vi "LWXPS_GetType.vi"(3 "LabVIEW error IN":errorcluster, 5 "XPS Reference IN":refnum<k24>) -> (0 "LabVIEW error OUT":errorcluster, 1 "Type":refnum<k24>, 2 "XPS Reference OUT":refnum<k24>)   [LabVIEW 2014]
uses:
  D:/XPSQ8_LabView_Library/Development/Source/Dll/Newport.XPS.CommandInterface.dll
  Dll/Newport.XPS.CommandInterface.dll
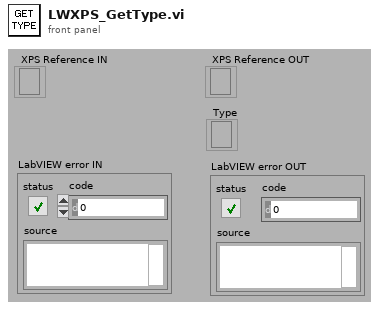
[diagram p1: front panel]
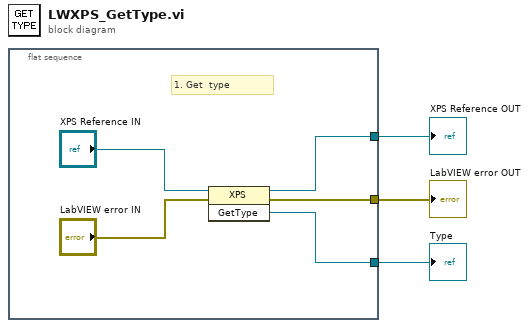
[diagram p0: block diagram]
diagram:
  n1 = flat-sequence {
    tunnel: [w7] -> w3
    tunnel: [w6] -> w2
    tunnel: [w4] -> w1
    frame #0 {
      # "1. Get  type"
      n2 = invoke class="XPS" method="GetType"(reference="XPS Reference IN", error in="LabVIEW error IN") -> (reference out=w7:refnum<k24>, error out=w6:errorcluster, "GetType"=w4:refnum<k24>)  [unwired: 1 in]
    }
  }
  "XPS Reference OUT" <- w3
  "LabVIEW error OUT" <- w2
  "Type" <- w1
